vi "Delete_Statuses_from_Processed_Subtracks-1.vi"(4 "error IN":errorcluster, 7 "[IN] Processed Tracks":T1(array[cluster])) -> (0 "error OUT":errorcluster, 3 "[OUT] Tracks":cluster{"Track":dbl[], "Start Pos":i32}[](array[cluster]))   [LabVIEW 2013]
doc: "SubVI deletes the statuses of points after tracking (unnecessary info)"
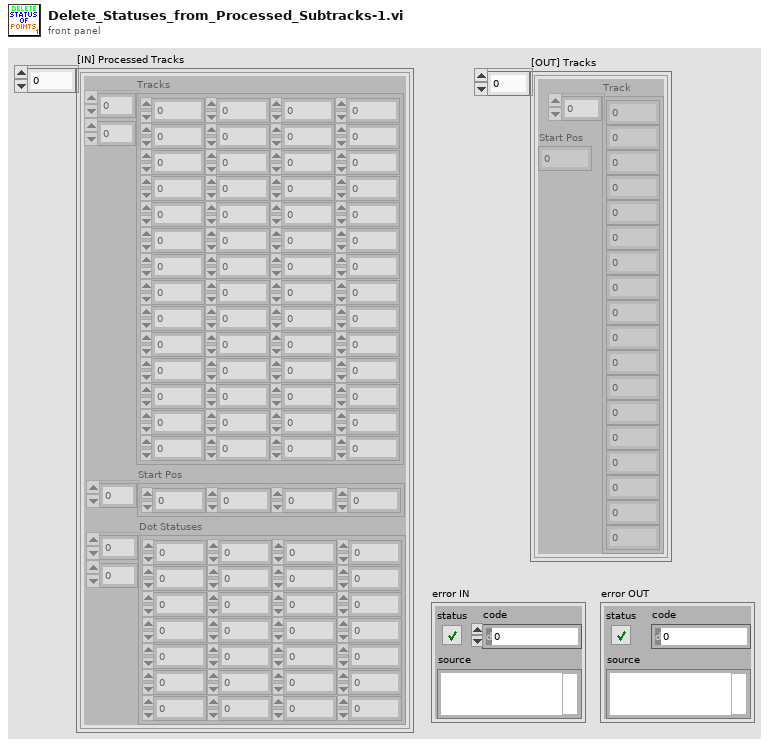
[diagram p1: front panel]
types:
  T1 = cluster{"Tracks":dbl[][], "Start Pos":i32[], "Dot Statuses":i16[][]}[]
  T2 = cluster{"Tracks":dbl[][], "Start Pos":i32[], "Dot Statuses":i16[][]}
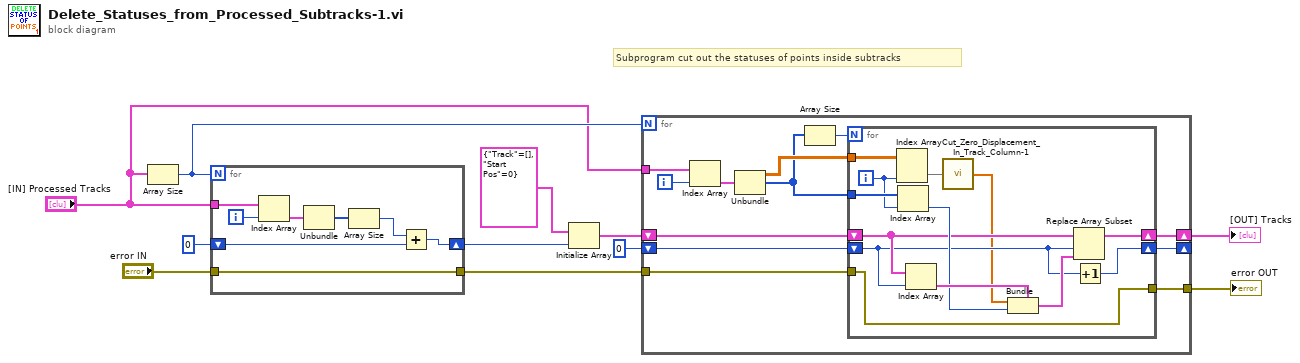
[diagram p0: block diagram]
diagram:
  # "Subprogram cut out the statuses of points inside subtracks"
  n1 = Array Size(array="[IN] Processed Tracks") -> (size(s)=w9:i32)
  n2 = for {
    N: w9 -> [_]
    tunnel: "[IN] Processed Tracks" -> [w18]
    tunnel: "error IN" -> [w16]
    tunnel: [w16] -> w3
    shift-right: [w12] -> w6
    shift-left: 0 -> [w13]
    i -> [w17]
    n3 = Index Array(array=w18, index=w17) -> (element=w19:T2)
    n4 = Unbundle(w19) -> ("Start Pos"=w15:i32[])  [unwired: 2 out]
    n5 = Array Size(array=w15) -> (size(s)=w14:i32)
    n6 = Add(x=w14, y=w13) -> (x+y=w12:i32)
  }
  n7 = Initialize Array(cluster{"Track":dbl[], "Start Pos":i32} {"Track"=[], "Start Pos"=0} ("element"), w6) -> (w5:cluster{"Track":dbl[], "Start Pos":i32}[])
  n8 = for {
    N: w9 -> [_]
    tunnel: "[IN] Processed Tracks" -> [w31]
    shift-right: [w23] -> w1
    shift-left: w5 -> [w25]
    shift-right: [w22] -> _
    shift-left: 0 -> [w24]
    tunnel: w3 -> [w21]
    tunnel: [w20] -> w2
    i -> [w30]
    n9 = Index Array(array=w31, index=w30) -> (element=w29:T2)
    n10 = Unbundle(w29) -> ("Tracks"=w27:dbl[][], "Start Pos"=w26:i32[])  [unwired: 1 out]
    n11 = Array Size(array=w26) -> (size(s)=w28:i32)
    n12 = for {
      N: w28 -> [_]
      tunnel: w27 -> [w44]
      tunnel: w26 -> [w43]
      shift-right: [w38] -> w23
      shift-left: w25 -> [w39]
      shift-right: [w35] -> w22
      shift-left: w24 -> [w36]
      tunnel: w21 -> [w34]
      tunnel: [w34] -> w20
      i -> [w42]
      n13 = Index Array(array=w44, index (col)=w42) -> (element=w33:dbl[])  [unwired: 1 in]
      n14 = Index Array(array=w43, index=w42) -> (element=w40:i32)
      n15 = Index Array(array=w39, index=w36) -> (element=w41:cluster{"Track":dbl[], "Start Pos":i32})
      n16 = call "Cut_Zero_Displacement_In_Track_Column-1.vi"("[IN] Track in column"=w33) -> ("[OUT] Track in column\nwithout zero points"=w32:dbl[])
      n17 = Bundle(cluster=w41, "Track"=w32, "Start Pos"=w40) -> (w37:cluster{"Track":dbl[], "Start Pos":i32})
      n18 = Replace Array Subset(array=w39, new element=w37, index=w36) -> (w38:cluster{"Track":dbl[], "Start Pos":i32}[])
      n19 = Increment(x=w36) -> (x+1=w35:i32)
    }
  }
  "error OUT" <- w2
  "[OUT] Tracks" <- w1
